vi "Create All Message Queues.vi"(8 "error in (no error)":errorcluster, 10 "DUT":string, 11 "This VI":refnum<vi>) -> (0 "error out":errorcluster, 3 "Message Queues out":T1)   [LabVIEW 2024, in "Keysight_34461a.lvlib" / "Message Queue.lvlib"]
doc: "This VI creates and initializes all the message queues for your application. If your application requires more than one message queue, right-click the \"Message Queues\" constant above and select Open Type Def. Add the new Message Queue(s) to the type definition, then initialize them in this VI."
uses:
  Message Queue.lvlib
  All Message Queues.ctl
  Enqueue Message (Single).vi
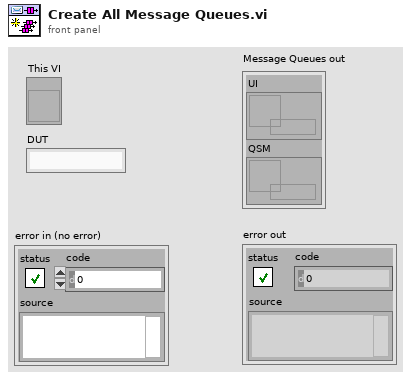
[diagram p1: front panel]
types:
  T1 = typedef "Keysight_34461a.lvlib/Message Queue.lvlib/All Message Queues.ctl" = cluster{"UI":refnum<queue>, "QSM":refnum<queue>}
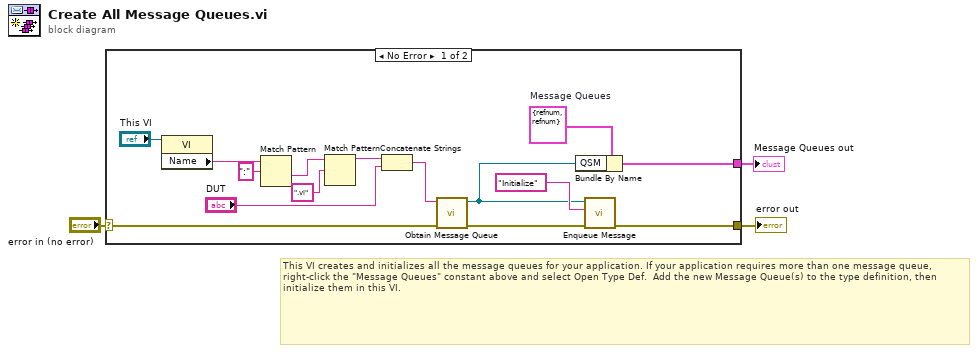
[diagram p0: block diagram]
diagram:
  # "This VI creates and initializes all the message queues for your application. If your application requires more than one message queue, right-click the \"Message Queues\" constant above and select Open Type Def.  Add the new Message Queue(s) to the type definition, then initialize them in this VI."
  n1 = case shown="No Error" "error in (no error)" {
    selector: "error in (no error)" -> [w15 w19]
    tunnel: [w18 w19] -> w3
    tunnel: [w16 _] -> w2
    frame No Error {
      w17 = T1 {"UI"=refnum, "QSM"=refnum}  # Message Queues
      n2 = property class="VI"(reference="This VI") -> ("Name"=w5:string)  [unwired: 1 in, 2 out]
      n3 = Match Pattern(string=w5, regular expression=":") -> (after substring=w9:string)  [unwired: 1 in, 3 out]
      n4 = Match Pattern(string=w9, regular expression=".vi") -> (before substring=w7:string)  [unwired: 1 in, 3 out]
      n5 = Concatenate Strings(w7, "DUT") -> (w4:string)
      n6 = call "Obtain Message Queue.vi"("error in (no error)"=w15, "Queue Name"=w4) -> ("error out"=w14:errorcluster, "Message Queue"=w12:refnum<queue>)  [unwired: 8 in]
      n7 = Bundle By Name(cluster=w17, "QSM"=w12) -> (w16:T1)
      n8 = call-poly "Enqueue Message.vi"("error in (no error)"=w14, "Message"="Initialize", "Message Queue"=w12) -> ("error out"=w18:errorcluster)  [unwired: 7 in, 1 out]
    }
    frame Error {
    }
  }
  "Message Queues out" <- w2
  "error out" <- w3
